vi "Global 1.vi"() -> ()   [LabVIEW 2018]
panel:
  in  "Numeric":dbl
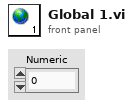
[diagram p1: front panel]
diagram:
